vi "test_Set and Get Propagation.vi"(8 "error in (no error)":errorcluster, 11 "TestCase in":refnum<class "Scan Engine Scripting API Custom Device Unit Tests.lvclass">) -> (0 "error out":errorcluster, 3 "TestCase out":refnum<class "Scan Engine Scripting API Custom Device Unit Tests.lvclass">)   [LabVIEW 2017, in "Scan Engine Scripting API Custom Device Unit Tests.lvclass"]
uses:
  Scan Engine Scripting API Custom Device Unit Tests.lvclass
  Scripting/Modules/Mode Classes/Controls/thermocouple channel settings.ctl
  Scripting/Modules/Channel Classes/Thermocouple Channel/Thermocouple Type.ctl
  Scripting/Modules/Channel Classes/Thermocouple Channel/Measurement Units.ctl
  Scripting/Modules/NI 9212/NI 9212 Settings.ctl
  Scripting/Modules/NI 9212/NI 9212 Conversion Time.ctl
  Scan Engine Scripting API Custom Device Unit Tests.lvclass/Scan Engine Scripting API Custom Device Unit Tests.ctl
  Type Defs/Main Settings.ctl
  Type Defs/Local Chassis Settings.ctl
  Scripting/Modules/NI 9212/NI 9212.lvclass
  C:/dev/niveristand-scan-engine-ethercat-custom-device/Custom Device Source/Scripting/Modules/Module/Module.lvclass
  260a9b95-26cc-4b9e-8ea8-5773fb04867b.vi
  Utility/Set Error.vi
  <vilib>/Utility/error.llb/Clear Errors.vi
  Scripting/Utility/Convert Slot Configuration to 9212.vi
  Scripting/Utility/Convert Slot Configuration to 9213.vi
  Modules.lvlibp/SD Module/SD Module.lvclass
  C:/dev/niveristand-scan-engine-ethercat-custom-device/Custom Device Source/Modules.lvlibp/RSI Module/RSI Module.lvclass
  Scripting/Modules/NI 9213/NI 9213.lvclass
  Scripting/Modules/NI 9224/NI 9224.lvclass
  Scripting/Modules/NI 9228/NI 9228.lvclass
  Modules.lvlibp/RSI Module/Read Module Page Property.vi
  Modules.lvlibp/RSI Module/Read Model.vi
  Scripting/Utility/Convert Module Model to Module Class.vi
  Modules.lvlibp/SD Module/Read DIO mode.vi
  Modules.lvlibp/RSI Module/Read Channels.vi
  Scripting/Utility/Convert to DI Module.vi
  Scripting/Utility/Convert to DO Module.vi
  Scripting/Utility/Convert to CI PWM Module.vi
  Scripting/Utility/Convert to CDO Module.vi
  Scripting/Utility/Convert to PWM Module.vi
  Globals/Error Strings.vi
  Scripting/Utility/Get Channel Names and Default Values for Slot.vi
  Scripting/Modules/NI 9213/Create NI 9213.vi
  Scripting/Utility/Convert to AI Module.vi
  Scripting/Utility/Convert to AI Vrms Module.vi
  Scripting/Utility/Convert to AI Arms Module.vi
  Scripting/Utility/Convert to DIO Module.vi
  Scripting/Modules/Module/Module.lvclass
  Modules.lvlibp/9212/9212.lvclass
  Modules.lvlibp/9213/9213.lvclass
  Modules.lvlibp/9224/9224.lvclass
  <vilib>/addons/_JKI Toolkits/VI Tester/TestCase.llb/TestCase.lvclass
  Scripting/Scan Engine Scripting.lvlib
  Scan Engine Custom Device.lvlib
  Scripting/Modules/Channel Classes/Thermocouple Channel/Thermocouple Channel.lvclass
  C:/Program Files (x86)/National Instruments/LabVIEW 2017/vi.lib/addons/_JKI Toolkits/VI Tester/TestCase.llb/TestCase.lvclass
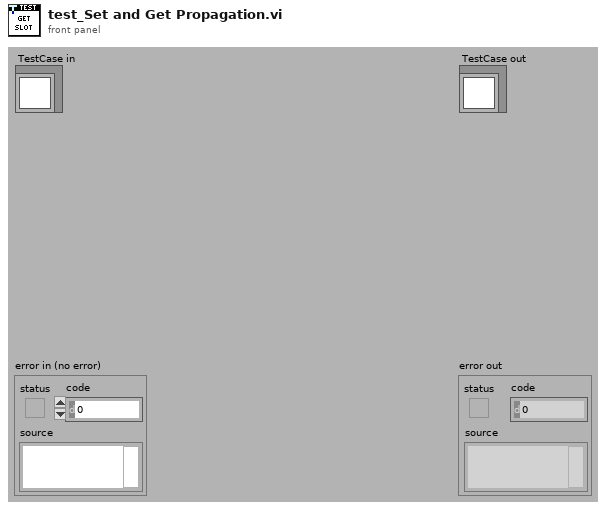
[diagram p1: front panel]
types:
  T1 = typedef "Scan Engine Scripting.lvlib/thermocouple channel settings.ctl" = cluster{"name":string, "default value":dbl, "thermocouple type":T2, "measurement units":T3}
  T2 = typedef "Scan Engine Scripting.lvlib/Thermocouple Channel.lvclass/Thermocouple Type.ctl" = enum16{"J", "K", "T", "E", "R", "S", "N", "B"}
  T3 = typedef "Scan Engine Scripting.lvlib/Thermocouple Channel.lvclass/Measurement Units.ctl" = enum16{"Raw Volts", "Degrees Kelvin", "Degrees Celsius", "Degrees Fahrenheit", "Degrees Rankine"}
  T4 = typedef "Scan Engine Custom Device.lvlib/Local Chassis Settings.ctl" = cluster{"name":string, "number of slots":i32}
  T5 = typedef "Scan Engine Custom Device.lvlib/Main Settings.ctl" = cluster{"sync to scan":bool, "scan engine decimation":u16, "delay after FPGA load (s)":u16}
  T6 = typedef "Scan Engine Scripting.lvlib/NI 9212.lvclass/NI 9212 Settings.ctl" = cluster{"conversion time":T7, "open thermocouple detection":bool}
  T7 = typedef "Scan Engine Scripting.lvlib/NI 9212.lvclass/NI 9212 Conversion Time.ctl" = enum16{"High Speed", "Best 60 Hz Rejection", "Best 50 Hz Rejection", "High Resolution"}
  T8 = typedef "Custom Device API.lvlib/Custom Device Item Ref.ctl" = u64
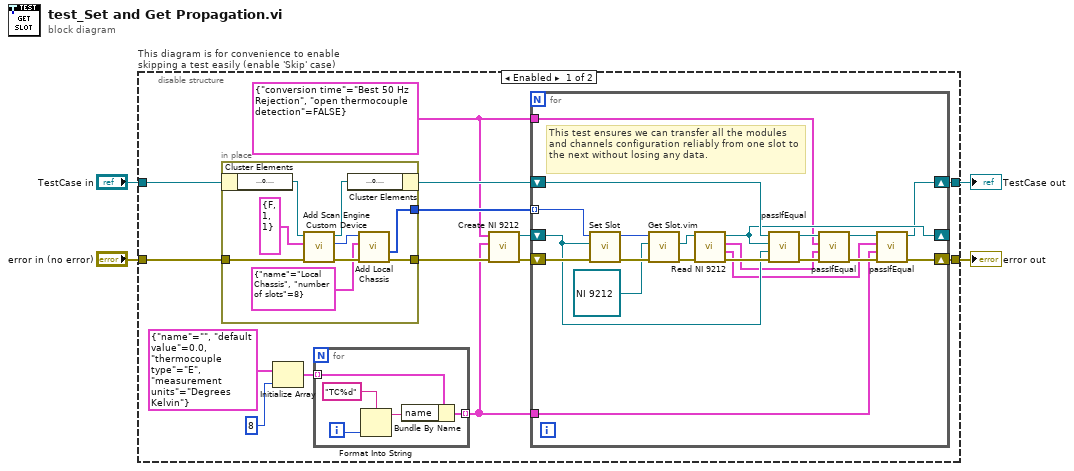
[diagram p0: block diagram]
diagram:
  n1 = disable-structure "This diagram is for convenience to enable skipping a test easily (enable 'Skip' case)" shown="Enabled" {
    disable-tunnel: "TestCase in" -> [w15 w57]
    disable-tunnel: [w17 w55] -> w1
    disable-tunnel: [w18 w56] -> w3
    disable-tunnel: "error in (no error)" -> [w16 w54]
    frame Enabled {
      w5 = T6 {"conversion time"=enum."Best 50 Hz Rejection", "open thermocouple detection"=FALSE} ("module settings")
      n2 = in-place {
        in-place-border: w16 -> [w32]
        in-place-border: [w25] -> w12
        in-place-border: [w24] -> w13
        n3 = in-place-cluster #1(w15) -> ("target ref"=w31:refnum<k24>)
        n4 = call "Add Scan Engine Custom Device.vi"("error in"=w32, "settings"=T5 {"sync to scan"=FALSE, "scan engine decimation"=1, "delay after FPGA load (s)"=1}, "target in"=w31) -> ("error out"=w28:errorcluster, "scan engine custom device ref"=w27:T8, "target out"=w30:refnum<k24>)  [unwired: 6 in]
        n5 = in-place-cluster #1("target ref"=w30) -> (w14:refnum<class "Scan Engine Scripting API Custom Device Unit Tests.lvclass">)
        n6 = call "Add Local Chassis.vi"("error in"=w28, "settings"=T4 {"name"="Local Chassis", "number of slots"=8}, "scan engine custom device ref in"=w27) -> ("error out"=w25:errorcluster, "slot refs"=w24:T8[])  [unwired: 4 in, 3 out]
      }
      n7 = Initialize Array(T1 {"name"="", "default value"=0.0, "thermocouple type"=enum."E", "measurement units"=enum."Degrees Kelvin"} ("channel settings"), 8 ("dimension size")) -> (w7:T1[])
      n8 = for {
        tunnel: w7 -> [w23] mode=indexing
        tunnel: [w19] -> w6 mode=indexing
        i -> [w22]
        n9 = Format Into String(format string="TC%d", w22) -> (resulting string=w20:string)  [unwired: 2 in, 1 out]
        n10 = Bundle By Name(cluster=w23, "name"=w20) -> (w19:T1)
      }
      n11 = call "Create NI 9212.vi"("error in"=w12, "channel settings"=w6, "module settings"=w5) -> ("error out"=w10:errorcluster, "NI 9212 out"=w11:refnum<class "NI 9212.lvclass">)  [unwired: 7 in]
      n12 = for {
        shift-right: [w37] -> w17
        shift-left: w14 -> [w52]
        tunnel: w13 -> [w47] mode=indexing
        shift-right: [w39] -> w18
        shift-left: w10 -> [w46]
        shift-right: [w45] -> _
        shift-left: w11 -> [w44]
        tunnel: w6 -> [w33]
        tunnel: w5 -> [w36]
        # "This test ensures we can transfer all the modules and channels configuration reliably from one slot to the next without losing any data."
        n13 = call "Set Slot.vi"("error in"=w46, "module"=w44, "slot ref in"=w47) -> ("error out"=w51:errorcluster, "slot ref out"=w50:T8)  [unwired: 7 in]
        n14 = call "Get Slot.vim"("error in"=w51, "module in"=refnum<class "NI 9212.lvclass"> refnum ("NI 9212 out"), "slot ref in"=w50) -> ("error out"=w49:errorcluster, "module"=w42:refnum<class "NI 9212.lvclass">)  [unwired: 5 in, 2 out]
        n15 = call "Read NI 9212.vi"("error in"=w49, "NI 9212 in"=w42) -> ("error out"=w48:errorcluster, "channel settings"=w34:T1[], "module settings"=w35:T6, "NI 9212 out"=w45:refnum<class "NI 9212.lvclass">)  [unwired: 6 in]
        n16 = call-dynamic "passIfEqual.vi"("error in (no error)"=w48, "y"=w44, "x"=w45, "TestCase in"=w52) -> ("error out"=w53:errorcluster, "TestCase out"=w40:refnum<class "Scan Engine Scripting API Custom Device Unit Tests.lvclass">)  [unwired: 6 in]
        n17 = call-dynamic "passIfEqual.vi"("error in (no error)"=w53, "y"=w35, "x"=w36, "TestCase in"=w40) -> ("error out"=w41:errorcluster, "TestCase out"=w38:refnum<class "Scan Engine Scripting API Custom Device Unit Tests.lvclass">)  [unwired: 6 in]
        n18 = call-dynamic "passIfEqual.vi"("error in (no error)"=w41, "y"=w33, "x"=w34, "TestCase in"=w38) -> ("error out"=w39:errorcluster, "TestCase out"=w37:refnum<class "Scan Engine Scripting API Custom Device Unit Tests.lvclass">)  [unwired: 6 in]
      }
    }
    frame Disabled {
      # "skip test result while test is under development"
      n19 = call <vilib>:"skip.vi"("error in (no error)"=w54, "TestCase in"=w57) -> ("error out"=w56:errorcluster, "TestCase out"=w55:refnum<class "Scan Engine Scripting API Custom Device Unit Tests.lvclass">)  [unwired: 8 in]
    }
  }
  "error out" <- w3
  "TestCase out" <- w1
